vi "reset_pattern.vi"(8 "error in (no error)":errorcluster, 11 "StimulatorDL090503Scaffold in":refnum<class "StimulatorDL090503Scaffold.lvclass">) -> (0 "error out":errorcluster, 3 "StimulatorDL090503Scaffold out":refnum<class "StimulatorDL090503Scaffold.lvclass">)   [LabVIEW 2010, in "StimulatorDL090503Scaffold.lvclass"]
uses:
  StimulatorDL090503Scaffold.lvclass
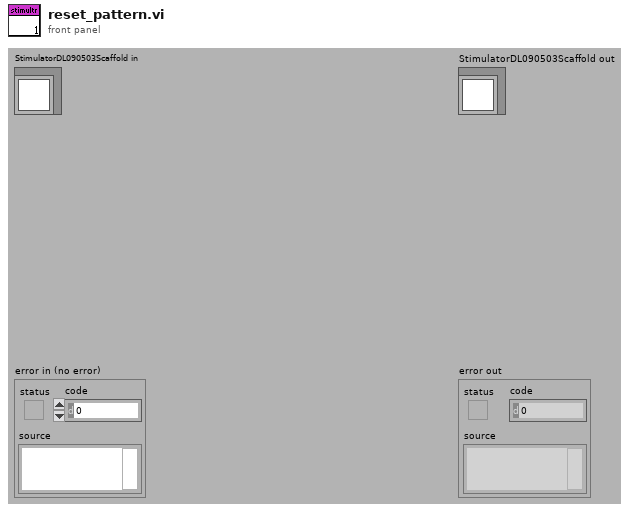
[diagram p1: front panel]
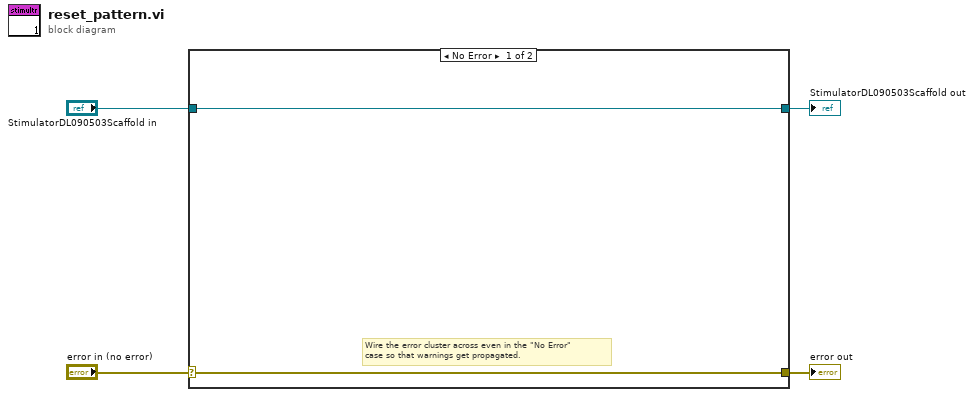
[diagram p0: block diagram]
diagram:
  n1 = case shown="No Error" "error in (no error)" {
    selector: "error in (no error)" -> [w5 w8]
    tunnel: [w5 w8] -> w3
    tunnel: [w6 w7] -> w1
    tunnel: "StimulatorDL090503Scaffold in" -> [w6 w7]
    frame No Error {
      # "Wire the error cluster across even in the \"No Error\"\ncase so that warnings get propagated."
    }
    frame Error {
    }
  }
  "error out" <- w3
  "StimulatorDL090503Scaffold out" <- w1
